vi "UHR-Fleezers Control (host) - 16.2.2v2.vi"() -> ()   [LabVIEW 2014] (continued)
                      n1466 = local write "Fl. High"(TRUE ("Fl. High")) -> ()
                      n1467 = Less?(x=w2263, y=w2254) -> (x < y?=w2261:bool)
                      n1468 = Or(x=w2260, y=w2261) -> (x .or. y?=w2256:bool)
                      n1469 = case shown="True" w2256 {
                        tunnel: w2259 -> [w2264 w2274]
                        tunnel: [w2264 w2273] -> w2258
                        tunnel: w2255 -> [_ w2272]
                        frame False {
                        }
                        frame True {
                          n1470 = flat-sequence {
                            tunnel: w2274 -> [w2280]
                            tunnel: w2272 -> [w2277]
                            tunnel: [w2279] -> w2271
                            tunnel: [w2278] -> w2270
                            tunnel: [w2277] -> w2269
                            tunnel: w2268 -> [w2276]
                            tunnel: [w2276] -> w2267
                            tunnel: w2266 -> [w2275]
                            tunnel: [w2275] -> w2265
                            tunnel: [w2351] -> w2273
                            tunnel: w2271 -> [w2351]
                            tunnel: w2270 -> [w2350]
                            tunnel: w2269 -> [w2349]
                            tunnel: w2267 -> [w2348]
                            tunnel: w2265 -> [w2347]
                            frame #0 {
                              n1471 = call <vilib>:"Beep.vi"() -> ()  [unwired: 12 in]
                              n1472 = local write "Waiting"(FALSE ("Waiting")) -> ()
                              n1473 = Increment(x=w2280) -> (x+1=w2279:i32)
                              n1474 = case shown="\"Image\"" w2277 {
                                tunnel: w2279 -> [_ w2285 _]
                                frame "Alarm", Default {
                                }
                                frame "Yank" {
                                n1475 = flat-sequence {
                                tunnel: w2285 -> [w2288]
                                tunnel: [w2287] -> w2284
                                tunnel: [w2286] -> w2283
                                tunnel: w2284 -> [w2298]
                                tunnel: w2283 -> [w2299]
                                frame #0 {
                                n1476 = local read "Yank Delay (s)"() -> (w2291:dbl)
                                n1477 = local read "N Array El"() -> (w2286:u8)
                                n1478 = Quotient & Remainder(x=w2288, y=w2286) -> (x-y*floor(x/y)=w2287:i32)  [unwired: 1 out]
                                n1479 = Multiply(x=w2291, y=1000.0) -> (x*y=w2289:dbl)
                                n1480 = Wait (ms)(milliseconds to wait=w2289) -> ()  [unwired: 1 out]
                                }
                                frame #1 {
                                n1481 = local read "Yank to which?"() -> (w2293:bool)
                                n1482 = local read "Random Choice"() -> (w2303:bool)
                                n1483 = local read "Yank to Trap Delta (MHz)"() -> (w2296:dbl[])
                                n1484 = local read "Yank to SP"() -> (w2297:dbl[])
                                n1485 = Random Number (0-1)() -> (number: 0 to 1=w2302:dbl)
                                n1486 = Multiply(x=w2299, y=w2302) -> (x*y=w2301:dbl)
                                n1487 = Round Toward -Infinity(1:w2301) -> (0:w2300:dbl)
                                n1488 = Select(t=w2300, s=w2303, f=w2298) -> (s? t:f=w2294:dbl)
                                n1489 = Select(t=w2296, s=w2293, f=w2297) -> (s? t:f=w2295:dbl[])
                                n1490 = Index Array(array=w2295, index=w2294) -> (element=w2292:dbl)
                                n1491 = case shown="True" w2293 {
                                tunnel: w2292 -> [w2304 w2331]
                                frame False {
                                n1492 = flat-sequence {
                                tunnel: w2304 -> [w2305]
                                frame #0 {
                                n1493 = property on="Trap Pos FB SP" class="DigNum (strict)"("Val(Sgnl)"=w2305) -> ()  [unwired: 2 in, 2 out]
                                }
                                frame #1 {
                                n1494 = Wait (ms)(milliseconds to wait=u32 700) -> ()  [unwired: 1 out]
                                }
                                frame #2 {
                                n1495 = local read "Action (%)"() -> (w2310:dbl)
                                n1496 = Absolute Value(x=w2310) -> (abs(x)=w2309:dbl)
                                n1497 = Greater?(x=w2309, y=70.0) -> (0:w2307:bool)
                                n1498 = property on="Remove Action Offset" class="Bool (strict)"("Val(Sgnl)"=w2307) -> ()  [unwired: 2 in, 2 out]
                                }
                                frame #3 {
                                n1499 = for {
                                N: 4 -> [_]
                                n1500 = flat-sequence {
                                frame #0 {
                                n1501 = Wait (ms)(milliseconds to wait=u32 500) -> ()  [unwired: 1 out]
                                }
                                frame #1 {
                                n1502 = local read "Action (%)"() -> (w2316:dbl)
                                n1503 = Absolute Value(x=w2316) -> (abs(x)=w2315:dbl)
                                n1504 = Greater?(x=w2315, y=70.0) -> (0:w2313:bool)
                                n1505 = property on="Remove Action Offset" class="Bool (strict)"("Val(Sgnl)"=w2313) -> ()  [unwired: 2 in, 2 out]
                                }
                                }
                                }
                                }
                                frame #4 {
                                n1506 = Wait (ms)(milliseconds to wait=u32 500) -> ()  [unwired: 1 out]
                                }
                                frame #5 {
                                n1507 = local read "Mean"() -> (w2324:dbl)
                                n1508 = Greater?(x=w2324, y=11.0) -> (0:w2318:bool)
                                n1509 = Not(x=w2318) -> (.not. x?=w2319:bool)
                                n1510 = And(x=w2319, y="Shift confocal") -> (x .and. y?=w2321:bool)
                                n1511 = And(x=w2318, y="Shift confocal") -> (x .and. y?=w2322:bool)
                                n1512 = case shown="True" w2322 {
                                frame False {
                                }
                                frame True {
                                n1513 = local read "Confocal Y 2 (V)"() -> (w2328:dbl)
                                n1514 = local read "Confocal X 2 (V)"() -> (w2327:dbl)
                                n1515 = property on="AO1" class="Slide (strict)"("Val(Sgnl)"=w2328) -> ()  [unwired: 2 in, 2 out]
                                n1516 = property on="AO2" class="Slide (strict)"("Val(Sgnl)"=w2327) -> ()  [unwired: 2 in, 2 out]
                                }
                                }
                                n1517 = case shown="True" w2321 {
                                frame False {
                                }
                                frame True {
                                n1518 = local read "Confocal Y 1 (V)"() -> (w2326:dbl)
                                n1519 = local read "Confocal X 1 (V)"() -> (w2325:dbl)
                                n1520 = property on="AO1" class="Slide (strict)"("Val(Sgnl)"=w2326) -> ()  [unwired: 2 in, 2 out]
                                n1521 = property on="AO2" class="Slide (strict)"("Val(Sgnl)"=w2325) -> ()  [unwired: 2 in, 2 out]
                                }
                                }
                                }
                                frame #6 {
                                n1522 = Wait (ms)(milliseconds to wait=u32 1500) -> ()  [unwired: 1 out]
                                }
                                frame #7 {
                                n1523 = property on="Rem fb disp offset" class="Bool (strict)"("Val(Sgnl)"=TRUE ("Value (Signaling)")) -> ()  [unwired: 2 in, 2 out]
                                }
                                }
                                }
                                frame True {
                                n1524 = flat-sequence {
                                tunnel: w2331 -> [w2332]
                                frame #0 {
                                n1525 = property on="Trap Delta (MHz)" class="DigNum (strict)"("Val(Sgnl)"=w2332) -> ()  [unwired: 2 in, 2 out]
                                }
                                frame #1 {
                                n1526 = Wait (ms)(milliseconds to wait=u32 500) -> ()  [unwired: 1 out]
                                }
                                frame #2 {
                                n1527 = local read "Shift confocal"() -> (w2338:bool)
                                n1528 = local read "Mean"() -> (w2340:dbl)
                                n1529 = Greater?(x=w2340, y=11.0) -> (0:w2337:bool)
                                n1530 = Not(x=w2337) -> (.not. x?=w2336:bool)
                                n1531 = And(x=w2336, y=w2338) -> (x .and. y?=w2334:bool)
                                n1532 = And(x=w2337, y=w2338) -> (x .and. y?=w2335:bool)
                                n1533 = case shown="True" w2335 {
                                frame False {
                                }
                                frame True {
                                n1534 = local read "Confocal Y 2 (V)"() -> (w2344:dbl)
                                n1535 = local read "Confocal X 2 (V)"() -> (w2343:dbl)
                                n1536 = property on="AO2" class="Slide (strict)"("Val(Sgnl)"=w2343) -> ()  [unwired: 2 in, 2 out]
                                n1537 = property on="AO1" class="Slide (strict)"("Val(Sgnl)"=w2344) -> ()  [unwired: 2 in, 2 out]
                                }
                                }
                                n1538 = case shown="True" w2334 {
                                frame False {
                                }
                                frame True {
                                n1539 = local read "Confocal X 1 (V)"() -> (w2341:dbl)
                                n1540 = local read "Confocal Y 1 (V)"() -> (w2342:dbl)
                                n1541 = property on="AO2" class="Slide (strict)"("Val(Sgnl)"=w2341) -> ()  [unwired: 2 in, 2 out]
                                n1542 = property on="AO1" class="Slide (strict)"("Val(Sgnl)"=w2342) -> ()  [unwired: 2 in, 2 out]
                                }
                                }
                                }
                                }
                                }
                                }
                                }
                                }
                                }
                                frame "Image" {
                                n1543 = property on="Confocal Image" class="Bool (strict)"("Val(Sgnl)"=TRUE ("Value (Signaling)")) -> ()  [unwired: 2 in, 2 out]
                                }
                              }
                              n1544 = local write "Fl. High"(FALSE ("Fl. High")) -> ()
                              n1545 = local read "Time (s)"() -> (w2278:dbl)
                            }
                            frame #1 {
                              n1546 = case shown="True" "Auto F Reset" {
                                tunnel: w2350 -> [_ w2355]
                                tunnel: w2349 -> [_ w2354]
                                tunnel: w2348 -> [_ w2353]
                                tunnel: w2347 -> [_ w2352]
                                frame False {
                                }
                                frame True {
                                n1547 = node-c288() -> (w2357:T28)  [unwired: 4 in]
                                n1548 = timed-loop {
                                timing: w2357 -> [_]
                                timing-out: [_] -> w2356
                                tunnel: w2355 -> [w2362]
                                tunnel: w2354 -> [w2361]
                                tunnel: w2353 -> [w2360]
                                tunnel: w2352 -> [w2359]
                                stop <- w2358 stop-if-true
                                n1549 = node-c288() -> ()  [unwired: 1 in, 1 out]
                                n1550 = local read "Fl. Delta Thresh. (kHz)"() -> (w2371:dbl)
                                n1551 = local read "APD to Watch"() -> (w2372:bool)
                                n1552 = local read "Delta Fl. 1"() -> (w2373:dbl)
                                n1553 = local read "Delta Fl. 2"() -> (w2374:dbl)
                                n1554 = local read "Fl. Triggered..."() -> (w2365:bool)
                                n1555 = local read "Stop All"() -> (w2366:bool)
                                n1556 = local read "Reset Force"() -> (w2364:bool)
                                n1557 = Multiply(x=w2371, y=1000.0) -> (x*y=w2369:dbl)
                                n1558 = Select(t=w2373, s=w2372, f=w2374) -> (s? t:f=w2368:dbl)
                                n1559 = Not(x=w2365) -> (.not. x?=w2363:bool)
                                n1560 = Greater?(x=w2368, y=w2369) -> (0:w2367:bool)
                                n1561 = Compound Arithmetic op=OR(w2367, w2366, w2363, w2364) -> (w2358:bool)
                                n1562 = case shown="True" w2358 {
                                tunnel: w2362 -> [_ w2378]
                                tunnel: w2361 -> [_ w2382]
                                tunnel: w2360 -> [_ w2381]
                                tunnel: w2359 -> [_ w2380]
                                frame False {
                                }
                                frame True {
                                n1563 = case shown="\"Yank\"" w2382 {
                                tunnel: w2381 -> [_ w2392]
                                tunnel: w2380 -> [_ w2390]
                                frame "Image", Default {
                                }
                                frame "Yank" {
                                n1564 = flat-sequence {
                                tunnel: [w2395] -> w2393
                                tunnel: w2392 -> [w2395]
                                tunnel: [w2394] -> w2391
                                tunnel: w2390 -> [w2394]
                                tunnel: w2393 -> [w2401]
                                tunnel: w2391 -> [w2399]
                                frame #0 {
                                n1565 = local read "Yank Delay (s)"() -> (w2398:dbl)
                                n1566 = Multiply(x=w2398, y=1000.0) -> (x*y=w2396:dbl)
                                n1567 = Wait (ms)(milliseconds to wait=w2396) -> ()  [unwired: 1 out]
                                }
                                frame #1 {
                                n1568 = local read "Yank to which?"() -> (w2400:bool)
                                n1569 = case shown="False" w2400 {
                                tunnel: w2401 -> [_ w2429]
                                tunnel: w2399 -> [w2402 _]
                                frame False {
                                n1570 = flat-sequence {
                                tunnel: w2402 -> [w2403]
                                frame #0 {
                                n1571 = property on="Trap Pos FB SP" class="DigNum (strict)"("Val(Sgnl)"=w2403) -> ()  [unwired: 2 in, 2 out]
                                }
                                frame #1 {
                                n1572 = Wait (ms)(milliseconds to wait=u32 700) -> ()  [unwired: 1 out]
                                }
                                frame #2 {
                                n1573 = local read "Action (%)"() -> (w2408:dbl)
                                n1574 = Absolute Value(x=w2408) -> (abs(x)=w2407:dbl)
                                n1575 = Greater?(x=w2407, y=70.0) -> (0:w2405:bool)
                                n1576 = property on="Remove Action Offset" class="Bool (strict)"("Val(Sgnl)"=w2405) -> ()  [unwired: 2 in, 2 out]
                                }
                                frame #3 {
                                n1577 = for {
                                N: 4 -> [_]
                                n1578 = flat-sequence {
                                frame #0 {
                                n1579 = Wait (ms)(milliseconds to wait=u32 500) -> ()  [unwired: 1 out]
                                }
                                frame #1 {
                                n1580 = local read "Action (%)"() -> (w2414:dbl)
                                n1581 = Absolute Value(x=w2414) -> (abs(x)=w2413:dbl)
                                n1582 = Greater?(x=w2413, y=70.0) -> (0:w2411:bool)
                                n1583 = property on="Remove Action Offset" class="Bool (strict)"("Val(Sgnl)"=w2411) -> ()  [unwired: 2 in, 2 out]
                                }
                                }
                                }
                                }
                                frame #4 {
                                n1584 = Wait (ms)(milliseconds to wait=u32 500) -> ()  [unwired: 1 out]
                                }
                                frame #5 {
                                n1585 = local read "Shift confocal"() -> (w2419:bool)
                                n1586 = local read "Mean"() -> (w2422:dbl)
                                n1587 = Greater?(x=w2422, y=11.0) -> (0:w2418:bool)
                                n1588 = Not(x=w2418) -> (.not. x?=w2417:bool)
                                n1589 = And(x=w2418, y=w2419) -> (x .and. y?=w2420:bool)
                                n1590 = And(x=w2417, y=w2419) -> (x .and. y?=w2416:bool)
                                n1591 = case shown="True" w2420 {
                                frame False {
                                }
                                frame True {
                                n1592 = local read "Confocal X 2 (V)"() -> (w2425:dbl)
                                n1593 = local read "Confocal Y 2 (V)"() -> (w2426:dbl)
                                n1594 = property on="AO2" class="Slide (strict)"("Val(Sgnl)"=w2425) -> ()  [unwired: 2 in, 2 out]
                                n1595 = property on="AO1" class="Slide (strict)"("Val(Sgnl)"=w2426) -> ()  [unwired: 2 in, 2 out]
                                }
                                }
                                n1596 = case shown="True" w2416 {
                                frame False {
                                }
                                frame True {
                                n1597 = local read "Confocal Y 1 (V)"() -> (w2424:dbl)
                                n1598 = local read "Confocal X 1 (V)"() -> (w2423:dbl)
                                n1599 = property on="AO1" class="Slide (strict)"("Val(Sgnl)"=w2424) -> ()  [unwired: 2 in, 2 out]
                                n1600 = property on="AO2" class="Slide (strict)"("Val(Sgnl)"=w2423) -> ()  [unwired: 2 in, 2 out]
                                }
                                }
                                }
                                frame #6 {
                                n1601 = Wait (ms)(milliseconds to wait=u32 1500) -> ()  [unwired: 1 out]
                                }
                                frame #7 {
                                n1602 = property on="Rem fb disp offset" class="Bool (strict)"("Val(Sgnl)"=TRUE ("Value (Signaling)")) -> ()  [unwired: 2 in, 2 out]
                                }
                                }
                                }
                                frame True {
                                n1603 = flat-sequence {
                                tunnel: w2429 -> [w2430]
                                frame #0 {
                                n1604 = property on="Trap Delta (MHz)" class="DigNum (strict)"("Val(Sgnl)"=w2430) -> ()  [unwired: 2 in, 2 out]
                                }
                                frame #1 {
                                n1605 = Wait (ms)(milliseconds to wait=u32 500) -> ()  [unwired: 1 out]
                                }
                                frame #2 {
                                n1606 = local read "Shift confocal"() -> (w2436:bool)
                                n1607 = local read "Mean"() -> (w2437:dbl)
                                n1608 = Greater?(x=w2437, y=11.0) -> (0:w2435:bool)
                                n1609 = And(x=w2435, y=w2436) -> (x .and. y?=w2433:bool)
                                n1610 = Not(x=w2435) -> (.not. x?=w2434:bool)
                                n1611 = And(x=w2434, y=w2436) -> (x .and. y?=w2432:bool)
                                n1612 = case shown="True" w2433 {
                                frame False {
                                }
                                frame True {
                                n1613 = local read "Confocal Y 2 (V)"() -> (w2442:dbl)
                                n1614 = local read "Confocal X 2 (V)"() -> (w2441:dbl)
                                n1615 = property on="AO1" class="Slide (strict)"("Val(Sgnl)"=w2442) -> ()  [unwired: 2 in, 2 out]
                                n1616 = property on="AO2" class="Slide (strict)"("Val(Sgnl)"=w2441) -> ()  [unwired: 2 in, 2 out]
                                }
                                }
                                n1617 = case shown="True" w2432 {
                                frame False {
                                }
                                frame True {
                                n1618 = local read "Confocal Y 1 (V)"() -> (w2440:dbl)
                                n1619 = local read "Confocal X 1 (V)"() -> (w2439:dbl)
                                n1620 = property on="AO2" class="Slide (strict)"("Val(Sgnl)"=w2439) -> ()  [unwired: 2 in, 2 out]
                                n1621 = property on="AO1" class="Slide (strict)"("Val(Sgnl)"=w2440) -> ()  [unwired: 2 in, 2 out]
                                }
                                }
                                }
                                }
                                }
                                }
                                }
                                }
                                }
                                }
                                n1622 = local read "Time (s)"() -> (w2377:dbl)
                                n1623 = Subtract(x=w2378, y=w2377) -> (x-y=w2389:dbl)
                                n1624 = Number To Decimal String(number=w2389, width (-)=i16 0) -> (decimal integer string=w2387:string)
                                n1625 = Concatenate Strings(w2387, " s fluorescence event") -> (w2384:string)
                                n1626 = local read "Messages"() -> (w2385:string)
                                n1627 = local write "Duration (s)"(w2389) -> ()
                                n1628 = call "Update messages.vi"("Message to add"=w2384, "Old message string"=w2385) -> ("New message string"=w2383:string)
                                n1629 = local write "Messages"(w2383) -> ()
                                n1630 = call <vilib>:"Beep.vi"() -> ()  [unwired: 12 in]
                                n1631 = local write "Reset Force"(FALSE ("Force Reset")) -> ()
                                n1632 = local write "Fl. High"(TRUE ("Fl. High")) -> ()
                                n1633 = local write "Waiting"(TRUE ("Waiting")) -> ()
                                }
                                }
                                n1634 = node-c288() -> ()  [unwired: 1 in, 1 out]
                                }
                                n1635 = node-c288(w2356) -> ()  [unwired: 1 out]
                                }
                              }
                            }
                          }
                          n1636 = local read "Trap Delta (MHz)"() -> (w2268:dbl)
                          n1637 = local read "Trap Pos FB SP"() -> (w2266:fxp<+/-,16,1>)
                        }
                      }
                    }
                    frame True {
                      n1638 = flat-sequence {
                        tunnel: w2453 -> [w2463]
                        tunnel: [w2463] -> w2457
                        tunnel: w2456 -> [w2462]
                        tunnel: [w2462] -> w2455
                        tunnel: [w2461] -> w2454
                        tunnel: w2452 -> [w2460]
                        tunnel: [w2459] -> w2451
                        tunnel: w2448 -> [w2458]
                        tunnel: [w2458] -> w2447
                        tunnel: w2457 -> [w2533]
                        tunnel: w2455 -> [w2532]
                        tunnel: w2454 -> [w2531]
                        tunnel: w2451 -> [w2530]
                        tunnel: w2447 -> [w2529]
                        tunnel: [w2530] -> w2450
                        frame #0 {
                          n1639 = call <vilib>:"Beep.vi"() -> ()  [unwired: 3 in, 9 out]
                          n1640 = local write "Waiting"(FALSE ("Waiting")) -> ()
                          n1641 = Increment(x=w2460) -> (x+1=w2459:u8)
                          n1642 = case shown="\"Yank\"" w2462 {
                            tunnel: w2459 -> [_ _ w2469]
                            frame "Image" {
                              n1643 = property on="Confocal Image" class="Bool (strict)"("Val(Sgnl)"=TRUE ("Value (Signaling)")) -> ()  [unwired: 2 in, 2 out]
                            }
                            frame "Alarm", Default {
                            }
                            frame "Yank" {
                              n1644 = flat-sequence {
                                tunnel: w2469 -> [w2472]
                                tunnel: [w2471] -> w2468
                                tunnel: ["N Array El"] -> w2467
                                tunnel: w2468 -> [w2486]
                                tunnel: w2467 -> [w2482]
                                frame #0 {
                                n1645 = Multiply(x="Yank Delay (s)", y=1000.0) -> (x*y=w2475:dbl)
                                n1646 = Quotient & Remainder(x=w2472, y="N Array El") -> (x-y*floor(x/y)=w2471:u8)  [unwired: 1 out]
                                n1647 = Wait (ms)(milliseconds to wait=w2475) -> ()  [unwired: 1 out]
                                }
                                frame #1 {
                                n1648 = Random Number (0-1)() -> (number: 0 to 1=w2483:dbl)
                                n1649 = Multiply(x=w2482, y=w2483) -> (x*y=w2481:dbl)
                                n1650 = Round Toward -Infinity(1:w2481) -> (0:w2480:dbl)
                                n1651 = Select(t=w2480, s="Random Choice", f=w2486) -> (s? t:f=w2484:dbl)
                                n1652 = Select(t="Yank to Trap Delta (MHz)", s="Yank to which?", f="Yank to SP") -> (s? t:f=w2477:dbl[])
                                n1653 = Index Array(array=w2477, index=w2484) -> (element=w2487:dbl)
                                n1654 = case shown="False" "Yank to which?" {
                                tunnel: w2487 -> [w2488 w2514]
                                frame False {
                                n1655 = flat-sequence {
                                tunnel: w2488 -> [w2489]
                                frame #0 {
                                n1656 = property on="Trap Pos FB SP" class="DigNum (strict)"("Val(Sgnl)"=w2489) -> ()  [unwired: 2 in, 2 out]
                                }
                                frame #1 {
                                n1657 = Wait (ms)(milliseconds to wait=u32 700) -> ()  [unwired: 1 out]
                                }
                                frame #2 {
                                n1658 = local read "Action (%)"() -> (w2494:dbl)
                                n1659 = Absolute Value(x=w2494) -> (abs(x)=w2493:dbl)
                                n1660 = Greater?(x=w2493, y=70.0) -> (0:w2491:bool)
                                n1661 = property on="Remove Action Offset" class="Bool (strict)"("Val(Sgnl)"=w2491) -> ()  [unwired: 2 in, 2 out]
                                }
                                frame #3 {
                                n1662 = for {
                                N: 4 -> [_]
                                n1663 = flat-sequence {
                                frame #0 {
                                n1664 = Wait (ms)(milliseconds to wait=u32 500) -> ()  [unwired: 1 out]
                                }
                                frame #1 {
                                n1665 = local read "Action (%)"() -> (w2500:dbl)
                                n1666 = Absolute Value(x=w2500) -> (abs(x)=w2499:dbl)
                                n1667 = Greater?(x=w2499, y=70.0) -> (0:w2497:bool)
                                n1668 = property on="Remove Action Offset" class="Bool (strict)"("Val(Sgnl)"=w2497) -> ()  [unwired: 2 in, 2 out]
                                }
                                }
                                }
                                }
                                frame #4 {
                                n1669 = local read "Shift confocal"() -> (w2504:bool)
                                n1670 = local read "Mean"() -> (w2507:dbl)
                                n1671 = Greater?(x=w2507, y=11.0) -> (0:w2503:bool)
                                n1672 = Not(x=w2503) -> (.not. x?=w2502:bool)
                                n1673 = And(x=w2502, y=w2504) -> (x .and. y?=w2501:bool)
                                n1674 = And(x=w2503, y=w2504) -> (x .and. y?=w2505:bool)
                                n1675 = case shown="True" w2505 {
                                frame False {
                                }
                                frame True {
                                n1676 = local read "Confocal X 2 (V)"() -> (w2510:dbl)
                                n1677 = local read "Confocal Y 2 (V)"() -> (w2511:dbl)
                                n1678 = property on="AO2" class="Slide (strict)"("Val(Sgnl)"=w2510) -> ()  [unwired: 2 in, 2 out]
                                n1679 = property on="AO1" class="Slide (strict)"("Val(Sgnl)"=w2511) -> ()  [unwired: 2 in, 2 out]
                                }
                                }
                                n1680 = case shown="True" w2501 {
                                frame False {
                                }
                                frame True {
                                n1681 = local read "Confocal X 1 (V)"() -> (w2508:dbl)
                                n1682 = local read "Confocal Y 1 (V)"() -> (w2509:dbl)
                                n1683 = property on="AO1" class="Slide (strict)"("Val(Sgnl)"=w2509) -> ()  [unwired: 2 in, 2 out]
                                n1684 = property on="AO2" class="Slide (strict)"("Val(Sgnl)"=w2508) -> ()  [unwired: 2 in, 2 out]
                                }
                                }
                                }
                                frame #5 {
                                n1685 = Wait (ms)(milliseconds to wait=u32 1500) -> ()  [unwired: 1 out]
                                }
                                frame #6 {
                                n1686 = property on="Rem fb disp offset" class="Bool (strict)"("Val(Sgnl)"=TRUE ("Value (Signaling)")) -> ()  [unwired: 2 in, 2 out]
                                }
                                }
                                }
                                frame True {
                                n1687 = flat-sequence {
                                tunnel: w2514 -> [w2515]
                                frame #0 {
                                n1688 = property on="Trap Delta (MHz)" class="DigNum (strict)"("Val(Sgnl)"=w2515) -> ()  [unwired: 2 in, 2 out]
                                }
                                frame #1 {
                                n1689 = Wait (ms)(milliseconds to wait=u32 500) -> ()  [unwired: 1 out]
                                }
                                frame #2 {
                                n1690 = local read "Shift confocal"() -> (w2519:bool)
                                n1691 = local read "Mean"() -> (w2517:dbl)
                                n1692 = Greater?(x=w2517, y=11.0) -> (0:w2520:bool)
                                n1693 = Not(x=w2520) -> (.not. x?=w2521:bool)
                                n1694 = And(x=w2521, y=w2519) -> (x .and. y?=w2523:bool)
                                n1695 = And(x=w2520, y=w2519) -> (x .and. y?=w2522:bool)
                                n1696 = case shown="True" w2522 {
                                frame False {
                                }
                                frame True {
                                n1697 = local read "Confocal Y 2 (V)"() -> (w2527:dbl)
                                n1698 = local read "Confocal X 2 (V)"() -> (w2526:dbl)
                                n1699 = property on="AO1" class="Slide (strict)"("Val(Sgnl)"=w2527) -> ()  [unwired: 2 in, 2 out]
                                n1700 = property on="AO2" class="Slide (strict)"("Val(Sgnl)"=w2526) -> ()  [unwired: 2 in, 2 out]
                                }
                                }
                                n1701 = case shown="True" w2523 {
                                frame False {
                                }
                                frame True {
                                n1702 = local read "Confocal X 1 (V)"() -> (w2524:dbl)
                                n1703 = local read "Confocal Y 1 (V)"() -> (w2525:dbl)
                                n1704 = property on="AO2" class="Slide (strict)"("Val(Sgnl)"=w2524) -> ()  [unwired: 2 in, 2 out]
                                n1705 = property on="AO1" class="Slide (strict)"("Val(Sgnl)"=w2525) -> ()  [unwired: 2 in, 2 out]
                                }
                                }
                                }
                                }
                                }
                                }
                                }
                              }
                            }
                          }
                          n1706 = local read "Time (s)"() -> (w2461:dbl)
                          "Fl. High" <- TRUE ("Yanking")
                        }
                        frame #1 {
                          n1707 = local read "Auto F Reset"() -> (w2528:bool)
                          n1708 = case shown="True" w2528 {
                            tunnel: w2533 -> [_ w2537]
                            tunnel: w2532 -> [_ w2536]
                            tunnel: w2531 -> [_ w2535]
                            tunnel: w2529 -> [_ w2534]
                            frame False {
                            }
                            frame True {
                              n1709 = node-c288() -> (w2539:T28)  [unwired: 4 out]
                              n1710 = timed-loop {
                                timing: w2539 -> [_]
                                timing-out: [_] -> w2538
                                tunnel: w2537 -> [w2557]
                                tunnel: w2536 -> [w2556]
                                tunnel: w2535 -> [w2555]
                                tunnel: w2534 -> [w2554]
                                stop <- w2540 stop-if-true
                                n1711 = node-c288() -> ()  [unwired: 2 out]
                                n1712 = local read "Fl. Delta Thresh. (kHz)"() -> (w2548:dbl)
                                n1713 = local read "Fl. Triggered..."() -> (w2553:bool)
                                n1714 = local read "Delta Fl. 1"() -> (w2544:dbl)
                                n1715 = local read "Delta Fl. 2"() -> (w2542:dbl)
                                n1716 = local read "Stop All"() -> (w2551:bool)
                                n1717 = local read "APD to Watch"() -> (w2543:bool)
                                n1718 = Select(t=w2544, s=w2543, f=w2542) -> (s? t:f=w2541:dbl)
                                n1719 = Not(x=w2553) -> (.not. x?=w2552:bool)
                                n1720 = Multiply(x=w2548, y=1000.0) -> (x*y=w2547:dbl)
                                n1721 = Negate(x=w2547) -> (-x=w2546:dbl)
                                n1722 = Less?(x=w2541, y=w2546) -> (x < y?=w2550:bool)
                                n1723 = Compound Arithmetic op=OR(w2550, w2551, w2552, "Reset Force") -> (w2540:bool)
                                n1724 = case shown="True" w2540 {
                                tunnel: w2557 -> [_ w2572]
                                tunnel: w2556 -> [_ w2571]
                                tunnel: w2555 -> [_ w2561]
                                tunnel: w2554 -> [_ w2563]
                                frame False {
                                }
                                frame True {
                                n1725 = local read "Time (s)"() -> (w2562:dbl)
                                n1726 = case shown="\"Yank\"" w2571 {
                                tunnel: w2572 -> [_ w2575]
                                tunnel: w2563 -> [_ w2573]
                                frame "Image", Default {
                                }
                                frame "Yank" {
                                n1727 = flat-sequence {
                                tunnel: [w2581] -> w2576
                                tunnel: w2575 -> [w2581]
                                tunnel: [w2577] -> w2574
                                tunnel: w2573 -> [w2577]
                                tunnel: w2576 -> [w2584]
                                tunnel: w2574 -> [w2582]
                                frame #0 {
                                n1728 = local read "Yank Delay (s)"() -> (w2580:dbl)
                                n1729 = Multiply(x=w2580, y=1000.0) -> (x*y=w2578:dbl)
                                n1730 = Wait (ms)(milliseconds to wait=w2578) -> ()  [unwired: 1 out]
                                }
                                frame #1 {
                                n1731 = local read "Yank to which?"() -> (w2583:bool)
                                n1732 = case shown="False" w2583 {
                                tunnel: w2584 -> [_ w2611]
                                tunnel: w2582 -> [w2585 _]
                                frame False {
                                n1733 = flat-sequence {
                                tunnel: w2585 -> [w2586]
                                frame #0 {
                                n1734 = property on="Trap Pos FB SP" class="DigNum (strict)"("Val(Sgnl)"=w2586) -> ()  [unwired: 2 in, 2 out]
                                }
                                frame #1 {
                                n1735 = Wait (ms)(milliseconds to wait=u32 700) -> ()  [unwired: 1 out]
                                }
                                frame #2 {
                                n1736 = local read "Action (%)"() -> (w2591:dbl)
                                n1737 = Absolute Value(x=w2591) -> (abs(x)=w2590:dbl)
                                n1738 = Greater?(x=w2590, y=70.0) -> (0:w2588:bool)
                                n1739 = property on="Remove Action Offset" class="Bool (strict)"("Val(Sgnl)"=w2588) -> ()  [unwired: 2 in, 2 out]
                                }
                                frame #3 {
                                n1740 = for {
                                N: 4 -> [_]
                                n1741 = flat-sequence {
                                frame #0 {
                                n1742 = Wait (ms)(milliseconds to wait=u32 500) -> ()  [unwired: 1 out]
                                }
                                frame #1 {
                                n1743 = local read "Action (%)"() -> (w2597:dbl)
                                n1744 = Absolute Value(x=w2597) -> (abs(x)=w2596:dbl)
                                n1745 = Greater?(x=w2596, y=70.0) -> (0:w2594:bool)
                                n1746 = property on="Remove Action Offset" class="Bool (strict)"("Val(Sgnl)"=w2594) -> ()  [unwired: 2 in, 2 out]
                                }
                                }
                                }
                                }
                                frame #4 {
                                n1747 = local read "Shift confocal"() -> (w2602:bool)
                                n1748 = local read "Mean"() -> (w2604:dbl)
                                n1749 = Greater?(x=w2604, y=11.0) -> (0:w2601:bool)
                                n1750 = Not(x=w2601) -> (.not. x?=w2600:bool)
                                n1751 = And(x=w2601, y=w2602) -> (x .and. y?=w2599:bool)
                                n1752 = And(x=w2600, y=w2602) -> (x .and. y?=w2598:bool)
                                n1753 = case shown="True" w2599 {
                                frame False {
                                }
                                frame True {
                                n1754 = local read "Confocal Y 2 (V)"() -> (w2608:dbl)
                                n1755 = local read "Confocal X 2 (V)"() -> (w2607:dbl)
                                n1756 = property on="AO2" class="Slide (strict)"("Val(Sgnl)"=w2607) -> ()  [unwired: 2 in, 2 out]
                                n1757 = property on="AO1" class="Slide (strict)"("Val(Sgnl)"=w2608) -> ()  [unwired: 2 in, 2 out]
                                }
                                }
                                n1758 = case shown="True" w2598 {
                                frame False {
                                }
                                frame True {
                                n1759 = local read "Confocal X 1 (V)"() -> (w2605:dbl)
                                n1760 = local read "Confocal Y 1 (V)"() -> (w2606:dbl)
                                n1761 = property on="AO1" class="Slide (strict)"("Val(Sgnl)"=w2606) -> ()  [unwired: 2 in, 2 out]
                                n1762 = property on="AO2" class="Slide (strict)"("Val(Sgnl)"=w2605) -> ()  [unwired: 2 in, 2 out]
                                }
                                }
                                }
                                frame #5 {
                                n1763 = Wait (ms)(milliseconds to wait=u32 1500) -> ()  [unwired: 1 out]
                                }
                                frame #6 {
                                n1764 = property on="Rem fb disp offset" class="Bool (strict)"("Val(Sgnl)"=TRUE ("Value (Signaling)")) -> ()  [unwired: 2 in, 2 out]
                                }
                                }
                                }
                                frame True {
                                n1765 = flat-sequence {
                                tunnel: w2611 -> [w2612]
                                frame #0 {
                                n1766 = property on="Trap Delta (MHz)" class="DigNum (strict)"("Val(Sgnl)"=w2612) -> ()  [unwired: 2 in, 2 out]
                                }
                                frame #1 {
                                n1767 = Wait (ms)(milliseconds to wait=u32 500) -> ()  [unwired: 1 out]
                                }
                                frame #2 {
                                n1768 = local read "Shift confocal"() -> (w2618:bool)
                                n1769 = local read "Mean"() -> (w2620:dbl)
                                n1770 = Greater?(x=w2620, y=11.0) -> (0:w2617:bool)
                                n1771 = Not(x=w2617) -> (.not. x?=w2616:bool)
                                n1772 = And(x=w2617, y=w2618) -> (x .and. y?=w2615:bool)
                                n1773 = And(x=w2616, y=w2618) -> (x .and. y?=w2614:bool)
                                n1774 = case shown="True" w2615 {
                                frame False {
                                }
                                frame True {
                                n1775 = local read "Confocal Y 2 (V)"() -> (w2624:dbl)
                                n1776 = local read "Confocal X 2 (V)"() -> (w2623:dbl)
                                n1777 = property on="AO2" class="Slide (strict)"("Val(Sgnl)"=w2623) -> ()  [unwired: 2 in, 2 out]
                                n1778 = property on="AO1" class="Slide (strict)"("Val(Sgnl)"=w2624) -> ()  [unwired: 2 in, 2 out]
                                }
                                }
                                n1779 = case shown="True" w2614 {
                                frame False {
                                }
                                frame True {
                                n1780 = local read "Confocal Y 1 (V)"() -> (w2622:dbl)
                                n1781 = local read "Confocal X 1 (V)"() -> (w2621:dbl)
                                n1782 = property on="AO2" class="Slide (strict)"("Val(Sgnl)"=w2621) -> ()  [unwired: 2 in, 2 out]
                                n1783 = property on="AO1" class="Slide (strict)"("Val(Sgnl)"=w2622) -> ()  [unwired: 2 in, 2 out]
                                }
                                }
                                }
                                }
                                }
                                }
                                }
                                }
                                }
                                }
                                n1784 = local read "Messages"() -> (w2570:string)
                                n1785 = Subtract(x=w2562, y=w2561) -> (x-y=w2568:dbl)
                                "Duration (s)" <- w2568
                                n1786 = Number To Decimal String(number=w2568, width (-)=i16 0) -> (decimal integer string=w2566:string)
                                n1787 = Concatenate Strings(w2566, " s fluorescence event." ("string")) -> (w2564:string)
                                n1788 = call "Update messages.vi"("Message to add"=w2564, "Old message string"=w2570) -> ("New message string"=w2569:string)
                                n1789 = local write "Reset Force"(FALSE ("Reset Force")) -> ()
                                n1790 = local write "Waiting"(TRUE ("Waiting")) -> ()
                                n1791 = local write "Messages"(w2569) -> ()
                                n1792 = local write "Fl. High"(FALSE ("Fl. High")) -> ()
                                n1793 = call <vilib>:"Beep.vi"() -> ()  [unwired: 3 in, 9 out]
                                }
                                }
                                n1794 = node-c288() -> ()  [unwired: 2 out]
                              }
                              n1795 = node-c288(w2538) -> ()  [unwired: 1 out]
                            }
                          }
                        }
                      }
                      n1796 = local read "Trap Delta (MHz)"() -> (w2453:dbl)
                      n1797 = local read "Trap Pos FB SP"() -> (w2448:fxp<+/-,16,1>)
                    }
                  }
                }
                frame #1 {
                  n1798 = local read "Stop All"() -> (w2634:bool)
                  n1799 = local read "Fl. Triggered..."() -> (w2632:bool)
                  n1800 = Not(x=w2632) -> (.not. x?=w2633:bool)
                  n1801 = Or(x=w2633, y=w2634) -> (x .or. y?=w2631:bool)
                }
              }
              n1802 = case shown="True" w2225 {
                frame False {
                }
                frame True {
                  n1803 = local read "Confocal Y 1 (V)"() -> (w2235:dbl)
                  n1804 = local read "Confocal X 1 (V)"() -> (w2234:dbl)
                  n1805 = property on="AO2" class="Slide (strict)"("Val(Sgnl)"=w2234) -> ()  [unwired: 2 in, 2 out]
                  n1806 = property on="AO1" class="Slide (strict)"("Val(Sgnl)"=w2235) -> ()  [unwired: 2 in, 2 out]
                }
              }
              n1807 = case shown="True" w2225 {
                frame False {
                }
                frame True {
                  w2233 = FALSE ("Fl. High")
                  n1808 = local write "Waiting"(w2233) -> ()
                  n1809 = local write "Fl. High"(w2233) -> ()
                }
              }
              n1810 = node-c288() -> ()  [unwired: 2 out]
            }
            n1811 = node-c288(w2223) -> ()  [unwired: 1 out]
          }
        }
      }
      event "Start assembly line": Value Change {
        n1812 = event-data() -> ()  [unwired: 7 out]
        n1813 = case shown="True" "Start assembly line" {
          tunnel: w2640 -> [_ w2641]
          frame False {
          }
          frame True {
            n1814 = flat-sequence {
              tunnel: w2641 -> [w2646]
              tunnel: [w2645] -> w2643
              tunnel: w2643 -> [w2677]
              tunnel: [w2676] -> w2642
              tunnel: w2642 -> [w2679]
              tunnel: w2641 -> [w2697]
              frame #0 {
                w2644 = TRUE ("Value (Signaling)")
                n1815 = property on="Green Laser ON" class="Bool (strict)"("Val(Sgnl)"=w2644) -> ()  [unwired: 2 in, 2 out]
                "AL Running" <- w2644
              }
              frame #1 {
                n1816 = node-c288() -> (w2648:T28)  [unwired: 4 in]
                n1817 = timed-loop {
                  timing: w2648 -> [_]
                  timing-out: [_] -> w2647
                  tunnel: w2646 -> [w2655]
                  tunnel: [w2649] -> w2645
                  stop <- w2651 stop-if-true
                  n1818 = node-c288() -> ()  [unwired: 1 in, 1 out]
                  n1819 = local read "APD 1 Rate (Hz)"() -> (w2650:dbl)
                  n1820 = Multiply(x="Cy3 Fl.  Thresh. (kHz)", y=1000.0) -> (x*y=w2658:dbl)
                  n1821 = Greater?(x=w2650, y=w2658) -> (0:w2654:bool)
                  n1822 = case shown="True" w2654 {
                    tunnel: w2655 -> [_ w2661]
                    tunnel: [TRUE ("Stage Moving") w2660] -> w2653
                    frame False {
                    }
                    frame True {
                      n1823 = flat-sequence {
                        tunnel: w2661 -> [w2666]
                        tunnel: [w2671] -> w2660
                        frame #0 {
                          n1824 = Multiply(x="AL Delay (s)", y=u32 1000) -> (x*y=w2663:u32)
                          n1825 = Wait (ms)(milliseconds to wait=w2663) -> ()  [unwired: 1 out]
                        }
                        frame #1 {
                          n1826 = property on="Green Laser ON" class="Bool (strict)"("Val(Sgnl)"=FALSE ("Value (Signaling)")) -> ()  [unwired: 2 in, 2 out]
                        }
                        frame #2 {
                          # "upper spot"
                          n1827 = local read "Saved Stage Positions"() -> (w2669:dbl[][])
                          n1828 = local write "Stage Moving"(TRUE ("Stage Moving")) -> ()
                          n1829 = call "move to saved stage position.vi"("Stage VISA resource name in"=w2666, "Position"=5, "Saved Stage Positions"=w2669) -> ("error out"=w2667:errorcluster)  [unwired: 1 in, 1 out]
                          n1830 = local write "Stage Control Serial Error"(w2667) -> ()
                        }
                        frame #3 {
                          w2671 = FALSE ("Stage Moving")
                          n1831 = call <vilib>:"Beep.vi"() -> ()  [unwired: 3 in, 9 out]
                          n1832 = local write "Stage Moving"(w2671) -> ()
                        }
                      }
                    }
                  }
                  n1833 = local read "Stop assembly line"() -> (w2649:bool)
                  n1834 = Not(x=w2653) -> (.not. x?=w2652:bool)
                  n1835 = node-c288() -> ()  [unwired: 1 in, 1 out]
                  n1836 = Or(x=w2652, y=w2649) -> (x .or. y?=w2651:bool)
                }
                n1837 = node-c288(w2647) -> ()  [unwired: 1 out]
              }
              frame #2 {
                n1838 = Not(x=w2677) -> (.not. x?=w2676:bool)
                n1839 = case shown="True" w2676 {
                  frame False {
                  }
                  frame True {
